vi "Write Year.vi"(8 "error in (no error)":errorcluster, 10 "Year":i32, 11 "Vehicle in":refnum<class "Vehicle.lvclass">) -> (0 "error out":errorcluster, 3 "Vehicle out":refnum<class "Vehicle.lvclass">)   [LabVIEW 2020, in "Vehicle.lvclass"]
uses:
  Vehicle.lvclass
  Vehicle.lvclass/Vehicle.ctl
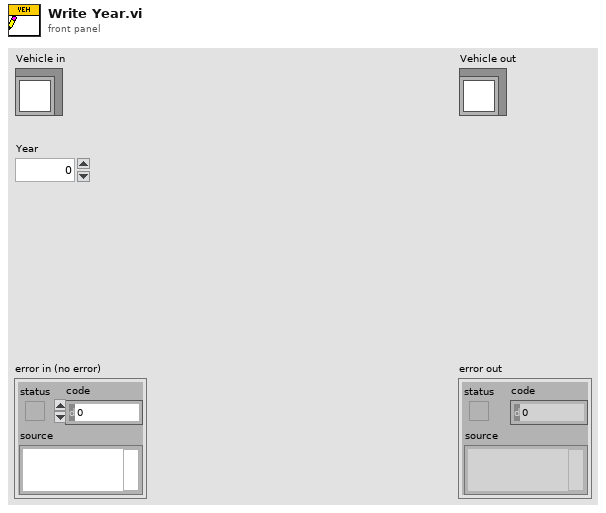
[diagram p1: front panel]
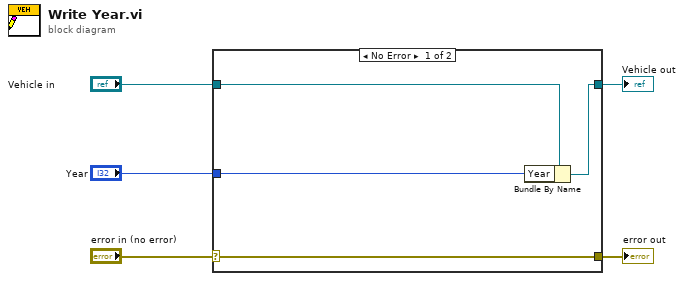
[diagram p0: block diagram]
diagram:
  n1 = case shown="No Error" "error in (no error)" {
    selector: "error in (no error)" -> [w9 w10]
    tunnel: [w9 w10] -> w4
    tunnel: [w7 w11] -> w2
    tunnel: "Vehicle in" -> [w8 w11]
    tunnel: "Year" -> [w6 _]
    frame No Error {
      n2 = Bundle By Name(cluster=w8, "Year"=w6) -> (w7:refnum<class "Vehicle.lvclass">)
    }
    frame Error {
    }
  }
  "error out" <- w4
  "Vehicle out" <- w2
